vi "CRYAna Spectrum.vi"(8 "EQ information":T2={"Stimulus EQ Curve"={"Name"="", "Curve"=[], "X data"=1, "Y data"=1, "Z data"=1, "X axis"=0, "Y axis"=1, "Z axis"=1, "X unit"="Hz", "Y unit"="", "Z unit"="deg.", "X dB ref"=1.0, "Y dB ref"=1.0, "Z dB ref"=1.0, "single val"=FALSE, "protected"=FALSE, "display X"=TRUE, "display Y"=TRUE, "display Z"=TRUE, "Test Info"="", "Step No."=0, "Plot Settings"={"Color"=0, "Interpolation"=0, "Point Style"=0, "Line Style"=0, "Point Color"=0, "Line Width"=0, "Bar Plot Style"=0, "Fill To"=0}, "AutoProtect"=FALSE}, "EQ"=FALSE, "EQ Rate"=0.0} {"EQ Rate" format="%.2f"; "Stimulus EQ Curve"."Z data" items=["dB", "Lin"]; "Stimulus EQ Curve"."X data" items=["dB", "Lin"]; "Stimulus EQ Curve"."Y data" items=["dB", "Lin"]; "Stimulus EQ Curve"."Z dB ref" format="%.1f"; "Stimulus EQ Curve"."Z axis" items=["Log", "Lin"]; "Stimulus EQ Curve"."X dB ref" format="%.1f"; "Stimulus EQ Curve"."X axis" items=["Log", "Lin"]; "Stimulus EQ Curve"."Y axis" items=["Log", "Lin"]; "Stimulus EQ Curve"."Y dB ref" format="%.1f"; "Stimulus EQ Curve"."Curve"."z" format="%.2f"; "Stimulus EQ Curve"."Curve"."y" format="%.2f"; "Stimulus EQ Curve"."Curve"."x" format="%.2f"}, 9 "Infor":T3={"window"=0, "Freq.Resolution"=10.0, "Overlap"=0.0, "Spectral Scaling"=0, "Sens In"=1.0} {"Sens In" format="%.2f"}, 10 "Wave Infor":cluster{"Fs":dbl, "Samples":dbl}={"Fs"=44100.0, "Samples"=0.0} {"Fs" min=1.0}, 11 "Signal":dbl[](array[numeric])) -> (1 "df":dbl format="%.2f", 2 "Spectrum X-axis":dbl[](array[numeric]) format="%.2f", 3 "Freq resp curves":cluster{cluster{dbl, dbl, dbl}[]}[](array[cluster]))   [LabVIEW 2013]
uses:
  Typedef Control/CRYData Cluster.ctl
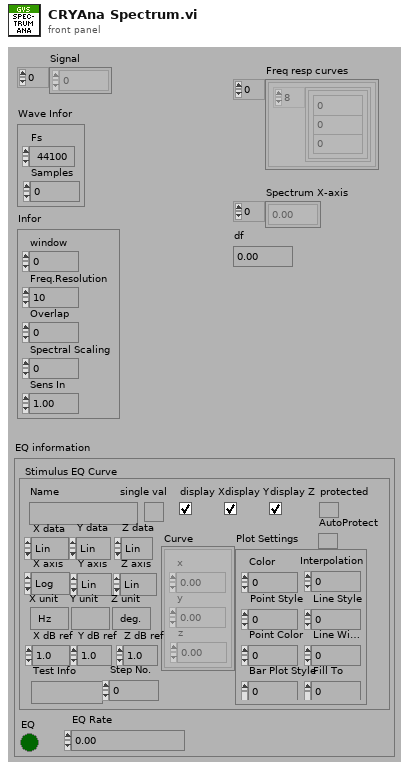
[diagram p1: front panel]
types:
  T1 = typedef "CRYData Cluster.ctl" = cluster{"Name":string, "Curve":cluster{"x":dbl, "y":dbl, "z":dbl}[], "X data":u16, "Y data":u16, "Z data":u16, "X axis":u16, "Y axis":u16, "Z axis":u16, "X unit":string, "Y unit":string, "Z unit":string, "X dB ref":dbl, "Y dB ref":dbl, "Z dB ref":dbl, "single val":bool, "protected":bool, "display X":bool, "display Y":bool, "display Z":bool, "Test Info":string, "Step No.":i32, "Plot Settings":cluster{"Color":u32, "Interpolation":u8, "Point Style":u8, "Line Style":u8, "Point Color":u32, "Line Width":u8, "Bar Plot Style":u8, "Fill To":i16}, "AutoProtect":bool}
  T2 = cluster{"Stimulus EQ Curve":T1, "EQ":bool, "EQ Rate":dbl}
  T3 = cluster{"window":u16, "Freq.Resolution":dbl, "Overlap":dbl, "Spectral Scaling":u16, "Sens In":dbl}
  T4 = cluster{"Fs":dbl, "Freq.Resolution":dbl, "Overlap":dbl, "window":u16}
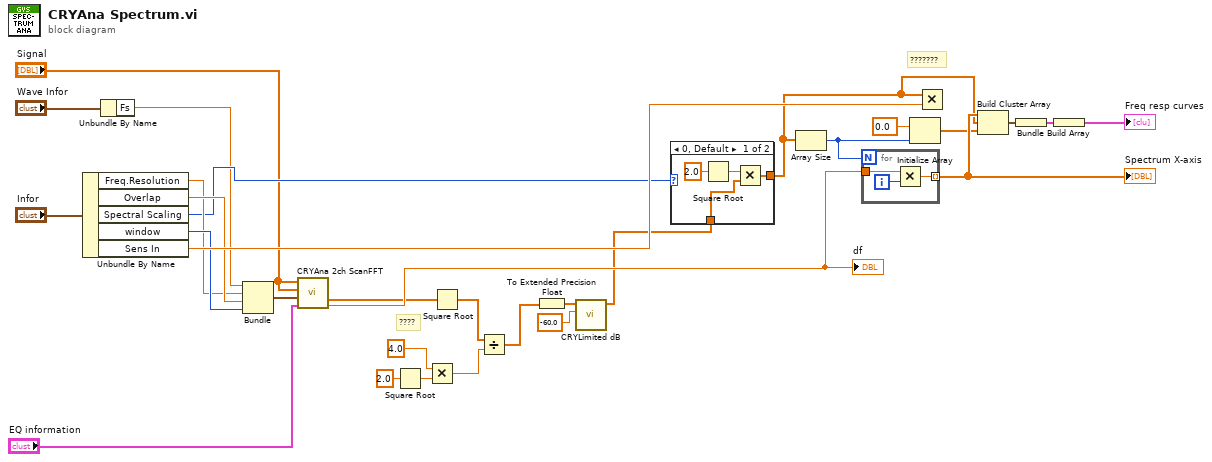
[diagram p0: block diagram]
diagram:
  # "????"
  # "???????"
  n1 = Unbundle By Name("Infor") -> ("Freq.Resolution"=w18:dbl, "Overlap"=w20:dbl, "Spectral Scaling"=w16:u16, "window"=w19:u16, "Sens In"=w22:dbl)
  n2 = Unbundle By Name("Wave Infor") -> ("Fs"=w12:dbl)
  n3 = Bundle("Fs"=w12, "Freq.Resolution"=w18, "Overlap"=w20, "window"=w19) -> (w21:T4)  [unwired: 1 in]
  n4 = call "CRYAna 2ch ScanFFT.vi"("EQ information"="EQ information", "In Parameter"=w21, "Response[y(t)]"="Signal", "Stimulus[x(t)]"="Signal") -> ("New dF(Hz)"=w11:dbl, "Gyy"=w10:dbl[])  [unwired: 4 in, 2 out]
  "df" <- w11
  n5 = Square Root(x=2.0) -> (sqrt(x)=w6:dbl)
  n6 = Multiply(x=4.0, y=w6) -> (x*y=w4:dbl)
  n7 = Square Root(x=w10) -> (sqrt(x)=w9:dbl[])
  n8 = Divide(x=w9, y=w4) -> (x/y=w8:dbl[])
  n9 = To Extended Precision Float(1:w8) -> (0:w13:ext[])
  n10 = call "CRYLimited dB.vi"("Dynamic(dB)"=-60.0, "Power spectrum"=w13) -> ("Limited spectrum"=w2:ext[])  [unwired: 9 in]
  n11 = case shown="0, Default" w16 {
    tunnel: w2 -> [w32 w35]
    tunnel: [w31 w35] -> w15
    frame 0, Default {
      n12 = Square Root(x=2.0) -> (sqrt(x)=w33:dbl)
      n13 = Multiply(x=w33, y=w32) -> (x*y=w31:ext[])
    }
    frame 1 {
    }
  }
  n14 = Array Size(array=w15) -> (size(s)=w24:i32)
  n15 = for {
    N: w24 -> [_]
    tunnel: [w37] -> w29 mode=indexing
    tunnel: w11 -> [w36]
    i -> [w38]
    n16 = Multiply(x=w36, y=w38) -> (x*y=w37:dbl)
  }
  "Spectrum X-axis" <- w29
  n17 = Initialize Array(0.0, w24) -> (w23:dbl[])
  n18 = Multiply(x=w15, y=w22) -> ()  [unwired: 1 out]
  n19 = Build Cluster Array(w29, w15, w23) -> (w30:cluster{dbl, "Log Out":ext, dbl}[])
  n20 = Bundle(w30) -> (w28:cluster{cluster{dbl, "Log Out":ext, dbl}[]})  [unwired: 1 in]
  n21 = Build Array(w28) -> (→"Freq resp curves":cluster{cluster{dbl, "Log Out":ext, dbl}[]}[])
